vi "serial read.vi"() -> ()   [LabVIEW 2020]
uses:
  <vilib>/Instr/_visa.llb/VISA Configure Serial Port (Instr).vi
panel:
  in  "SImpan Di Excel":bool
  out "read buffer":string
  out "Grafik Elektrokardiograf":i32(graph)
  in  "stop":bool
  in  "Port Kontroler":refnum<visa-resource-name>
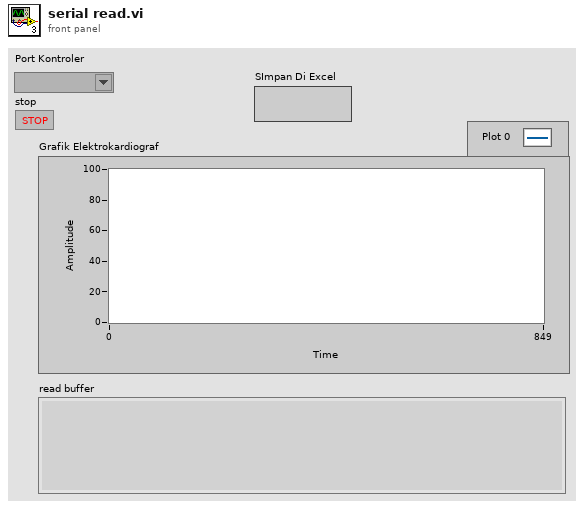
[diagram p1: front panel]
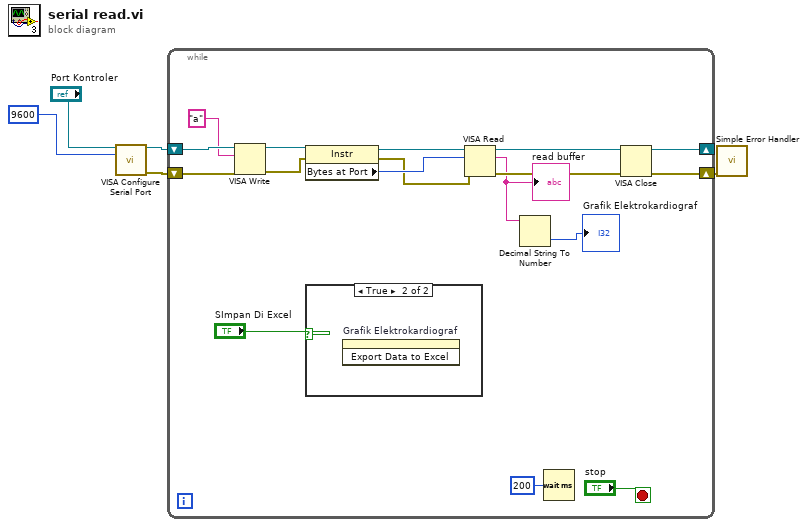
[diagram p0: block diagram]
diagram:
  n1 = call-poly "VISA Configure Serial Port"("VISA resource name"="Port Kontroler", "baud rate (9600)"=u32 9600) -> ("VISA resource name out"=w5:refnum<visa-resource-name>, "error out"=w4:errorcluster)  [unwired: 12 in]
  n2 = while {
    shift-right: [w14] -> w3
    shift-left: w5 -> [w22]
    shift-right: [w13] -> w2
    shift-left: w4 -> [w21]
    stop <- "stop" stop-if-true
    n3 = VISA Write(VISA resource name=w22, write buffer="a", error in (no error)=w21) -> (VISA resource name out=w20:refnum<visa-resource-name>, error out=w17:errorcluster)  [unwired: 1 out]
    n4 = property class="Instr"(reference=w20, error in=w17) -> (reference out=w19:refnum<visa-resource-name>, error out=w16:errorcluster, "Bytes at Port"=w18:u32)
    n5 = case shown="True" "SImpan Di Excel" {
      frame False {
      }
      frame True {
        n6 = invoke on="Grafik Elektrokardiograf" class="WFChart (strict)" method="Export Data to Excel"() -> ()  [unwired: 3 in, 3 out]
      }
    }
    n7 = VISA Read(VISA resource name=w19, byte count=w18, error in (no error)=w16) -> (VISA resource name out=w14:refnum<visa-resource-name>, read buffer=w11:string, error out=w13:errorcluster)  [unwired: 1 out]
    "read buffer" <- w11
    n8 = Decimal String To Number(string=w11) -> (number=→"Grafik Elektrokardiograf":i32)  [unwired: 2 in, 1 out]
    n9 = Wait (ms)(milliseconds to wait=u32 200) -> ()  [unwired: 1 out]
  }
  n10 = VISA Close(VISA resource name=w3, error in (no error)=w2) -> (error out=w1:errorcluster)
  n11 = call <vilib>:"Simple Error Handler.vi"("error in (no error)"=w1) -> ()  [unwired: 4 in, 5 out]
